vi "create_feature_studio.vi"(9 "wid":string, 10 "did":string, 11 "Name":string) -> (1 "path":string, 2 "payload":string, 3 "Method":string)   [LabVIEW 2019]
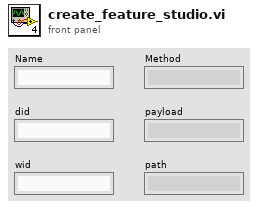
[diagram p1: front panel]
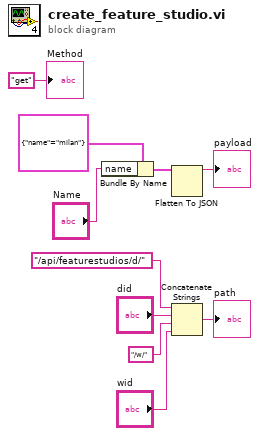
[diagram p0: block diagram]
diagram:
  n1 = Bundle By Name(cluster=cluster{"name":string} {"name"="milan"}, "name"="Name") -> (w2:cluster{"name":string})
  n2 = Flatten To JSON(anything=w2) -> (JSON string=→"payload":string)  [unwired: 2 in, 1 out]
  n3 = Concatenate Strings("/api/featurestudios/d/" ("payload"), "did", "/w/" ("string"), "wid") -> (→"path":string)
  "Method" <- "get" ("Method")
